vi "Vedio Input.vi"() -> ()   [LabVIEW 2021]
uses:
  <vilib>/userdefined/High Color/IMAQdx.ctl
  <vilib>/vision/driver/NI_Vision_Acquisition_Software.lvlib
panel:
  out "return value":i32
  in  "Numeric":i32
  in  "module path":path=path "D:/9th/LabVIEW/testing/function.py"
  in  "Python path":path=path "C:/Users/river/AppData/Local/Programs/Python/Python39/python.exe"
  in  "stop":bool
  out "Image":T1(plugin-control)
  in  "Session In":T2="cam0"
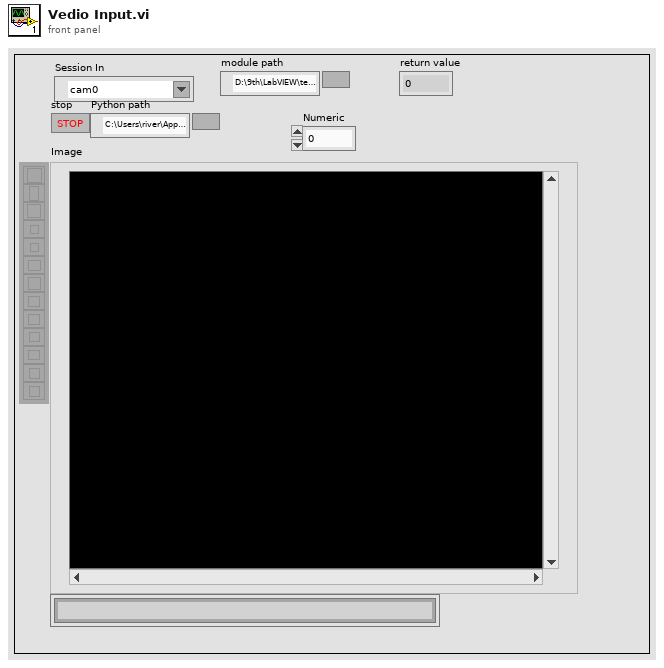
[diagram p1: front panel]
types:
  T1 = typedef "IMAQ Image.ctl" = refnum<image>
  T2 = typedef "IMAQdx.ctl" = refnum<k21>
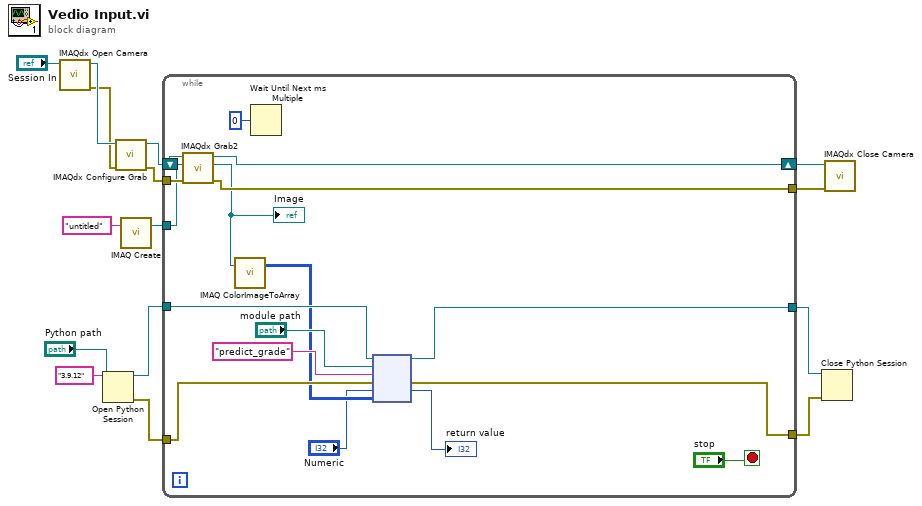
[diagram p0: block diagram]
diagram:
  n1 = call <vilib>:"IMAQdx Open Camera.vi"("Session In"="Session In") -> ("error out"=w13:errorcluster, "Session Out"=w14:T2)  [unwired: 9 in]
  n2 = Open Python Session(python version="3.9.12" ("Python version"), python path="Python path") -> (session out=w3:refnum<k35>, error out=w2:errorcluster)  [unwired: 1 in]
  n3 = call <vilib>:"IMAQdx Configure Grab.vi"("error in"=w13, "Session In"=w14) -> ("error out"=w11:errorcluster, "Session Out"=w12:T2)  [unwired: 8 in]
  n4 = call "IMAQ Create"("Image Name"="untitled") -> ("New Image"=w10:T1)  [unwired: 4 in, 1 out]
  n5 = while {
    tunnel: w11 -> [w31]
    tunnel: w10 -> [w30]
    shift-right: [w29] -> w8
    shift-left: w12 -> [w32]
    tunnel: [w28] -> w7
    tunnel: [w25] -> w4
    tunnel: w3 -> [w24]
    tunnel: w2 -> [w23]
    tunnel: [w22] -> w1
    stop <- "stop" stop-if-true
    n6 = call <vilib>:"IMAQdx Grab2.vi"("error in"=w31, "Image In"=w30, "Session In"=w32) -> ("error out"=w28:errorcluster, "Image Out"=w19:T1, "Session Out"=w29:T2)  [unwired: 5 in, 1 out]
    "Image" <- w19
    n7 = call "IMAQ ColorImageToArray"("Image"=w19) -> ("Image Pixels (U32)"=w18:u32[][])  [unwired: 3 in, 2 out]
    n8 = Wait Until Next ms Multiple(millisecond multiple=u32 0) -> ()  [unwired: 1 out]
    n9 = node(w24, "module path", "predict_grade" ("function name"), w23, "Numeric", w18) -> (w25:refnum<k35>, w22:errorcluster, →"return value":i32)  [unwired: 1 in, 2 out]
  }
  n10 = Close Python Session(session in=w4, error in=w1) -> ()  [unwired: 1 out]
  n11 = call <vilib>:"IMAQdx Close Camera.vi"("error in"=w7, "Session In"=w8) -> ()  [unwired: 9 in, 1 out]
